vi "Theta 3.vi"(9 "XYZ_ij":dbl[](array[numeric]), 10 "theta_4":dbl, 11 "6R Type 1 Serial Arm Class in":refnum<class "NI_Robotics_6R Type 1 Serial Arm Class.lvclass">) -> (1 "valid?":bool, 2 "theta_3":dbl, 3 "6R Type 1 Serial Arm Class out":refnum<class "NI_Robotics_6R Type 1 Serial Arm Class.lvclass">)   [LabVIEW 2017, in "NI_Robotics_6R Type 1 Serial Arm Class.lvclass"]
uses:
  <vilib>/robotics/Kinematics/Analytical/6R/Type 1/NI_Robotics_6R Type 1 Serial Arm Class.lvclass
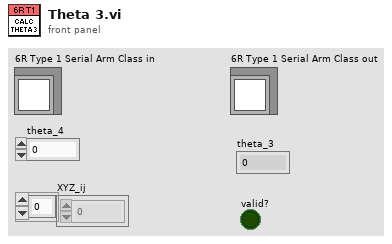
[diagram p1: front panel]
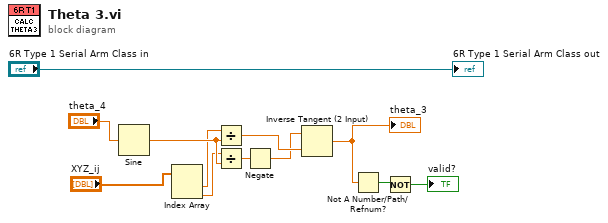
[diagram p0: block diagram]
diagram:
  n1 = Sine(x="theta_4") -> (sin(x)=w9:dbl)
  n2 = Index Array(array="XYZ_ij") -> (element #1=w7:dbl, element #2=w8:dbl)  [unwired: 2 in]
  n3 = Divide(x=w7, y=w9) -> (x/y=w12:dbl)
  n4 = Divide(x=w8, y=w9) -> (x/y=w10:dbl)
  n5 = Negate(x=w10) -> (-x=w11:dbl)
  n6 = Inverse Tangent (2 Input)(1:w12, 2:w11) -> (0:w1:dbl)
  "theta_3" <- w1
  n7 = Not A Number/Path/Refnum?(number/path/refnum=w1) -> (NaN/Path/Refnum?=w3:bool)
  n8 = Not(x=w3) -> (.not. x?=→"valid?":bool)
  "6R Type 1 Serial Arm Class out" <- "6R Type 1 Serial Arm Class in"
